vi "Eth Status Write Stop_com.vi"(7 "Status Reference":T1, 8 "error in (no error)":errorcluster, 10 "Stop":bool) -> (0 "error out":errorcluster)   [LabVIEW 2019, in "Eth Status.lvlib"]
uses:
  Eth Status.lvlib
  Ctl/ICPCON Status.ctl
  MB_TCP2/MB_TCP_State.ctl
  MB_TCP2/MB_TCP.lvclass
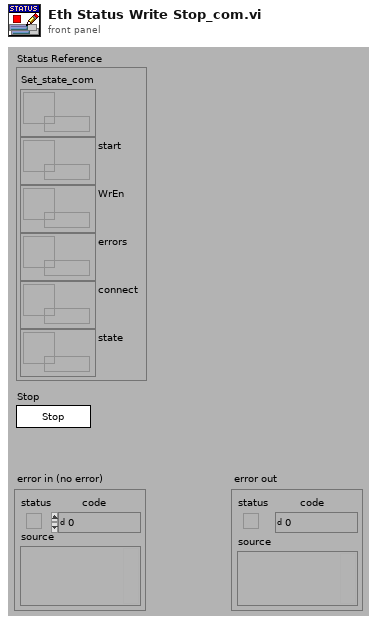
[diagram p1: front panel]
types:
  T1 = typedef "Eth Status.lvlib/ICPCON Status.ctl" = cluster{"Set_state_com":refnum<data-value>, "start":refnum<data-value>, "WrEn":refnum<data-value>, "errors":refnum<data-value>, "connect":refnum<data-value>, "state":refnum<data-value>}
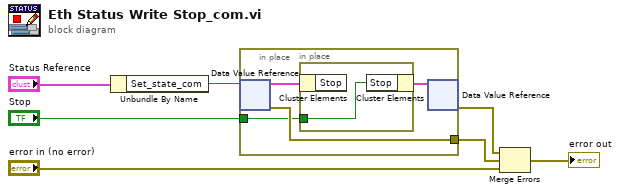
[diagram p0: block diagram]
diagram:
  n1 = Unbundle By Name("Status Reference") -> ("Set_state_com"=w1:refnum<data-value>)
  n2 = in-place {
    in-place-border: "Stop" -> [w9]
    in-place-border: [w11] -> w2
    n3 = in-place-dvr #1(w1) -> (w10:cluster{"Start":bool, "WrEn":bool, "Stop":bool}, w11:errorcluster)
    n4 = in-place {
      in-place-border: w9 -> [w12]
      n5 = in-place-cluster #2(w10) -> ()  [unwired: 1 out]
      n6 = in-place-cluster #2("Stop"=w12) -> (w8:cluster{"Start":bool, "WrEn":bool, "Stop":bool})
    }
    n7 = in-place-dvr #1(w8) -> (w3:errorcluster)  [unwired: 1 out]
  }
  n8 = Merge Errors(w3, w2, "error in (no error)") -> (→"error out":errorcluster)
